vi "Set Valve.vi"(8 "New State":bool=TRUE, 10 "Valve":T1) -> ()   [LabVIEW 2015]
uses:
  Valve Name Enum.ctl
  Valve Button Mapping Global Action.ctl
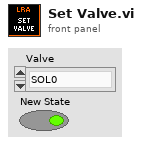
[diagram p1: front panel]
types:
  T1 = typedef "Valve Name Enum.ctl" = enum16{"SOL0", "COMP"}
  T2 = typedef "Valve Button Mapping Global Action.ctl" = enum16{"Get", "Set", "Init"}
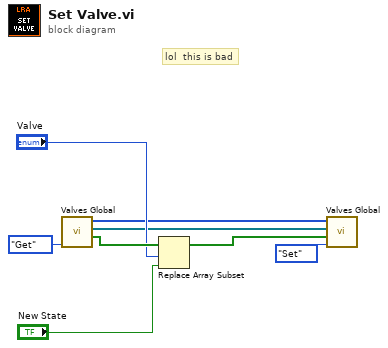
[diagram p0: block diagram]
diagram:
  # "lol  this is bad"
  n1 = call "Valves Global.vi"("Action"=Valve_Button_Mapping_Global_Action."Get") -> ("States"=w6:bool[], "Buttons"=w1:refnum<vi>[], "Valves"=w2:T1[])  [unwired: 7 in, 1 out]
  n2 = Replace Array Subset(array=w6, new element="New State", index="Valve") -> (w5:bool[])
  n3 = call "Valves Global.vi"("Action"=Valve_Button_Mapping_Global_Action."Set", "Valve States"=w5, "Valve Buttons"=w1, "Valves"=w2) -> ()  [unwired: 4 in, 4 out]
